vi "test enum2.vi"() -> ()   [LabVIEW 2020]
uses:
  OneDrive/_WorkingOn/Transformer-Project/Transformer/instr.lib/Ossila-X200-SMU-Driver/Public/Typedef/SMU OSR.ctl
  482ffdba-febc-40e4-8491-b362d5e89764.vi
  <userlib>/_NEVSTOP/Communicable State Machine(CSM)/addons/API-String-Arugments-Support/_Support/Convert API String Arguments to Data(variant).vi
  OneDrive/_WorkingOn/Transformer-Project/Transformer/instr.lib/Ossila-X200-SMU-Driver/Ossila X200 SMU.lvclass
panel:
  out "data 2":T1=enum."32768"
  out "Data":T1=enum."32768"
  out "data":T1=enum."32768"
  in  "element":string="4096"
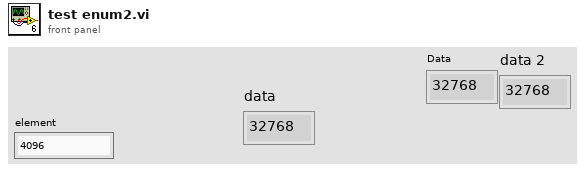
[diagram p1: front panel]
types:
  T1 = typedef "Ossila X200 SMU Instr.lvlib/Ossila X200 SMU.lvclass/SMU OSR.ctl" = enum16{"128", "256", "512", "1024", "2048", "4096", "8192", "16384", "32768"}
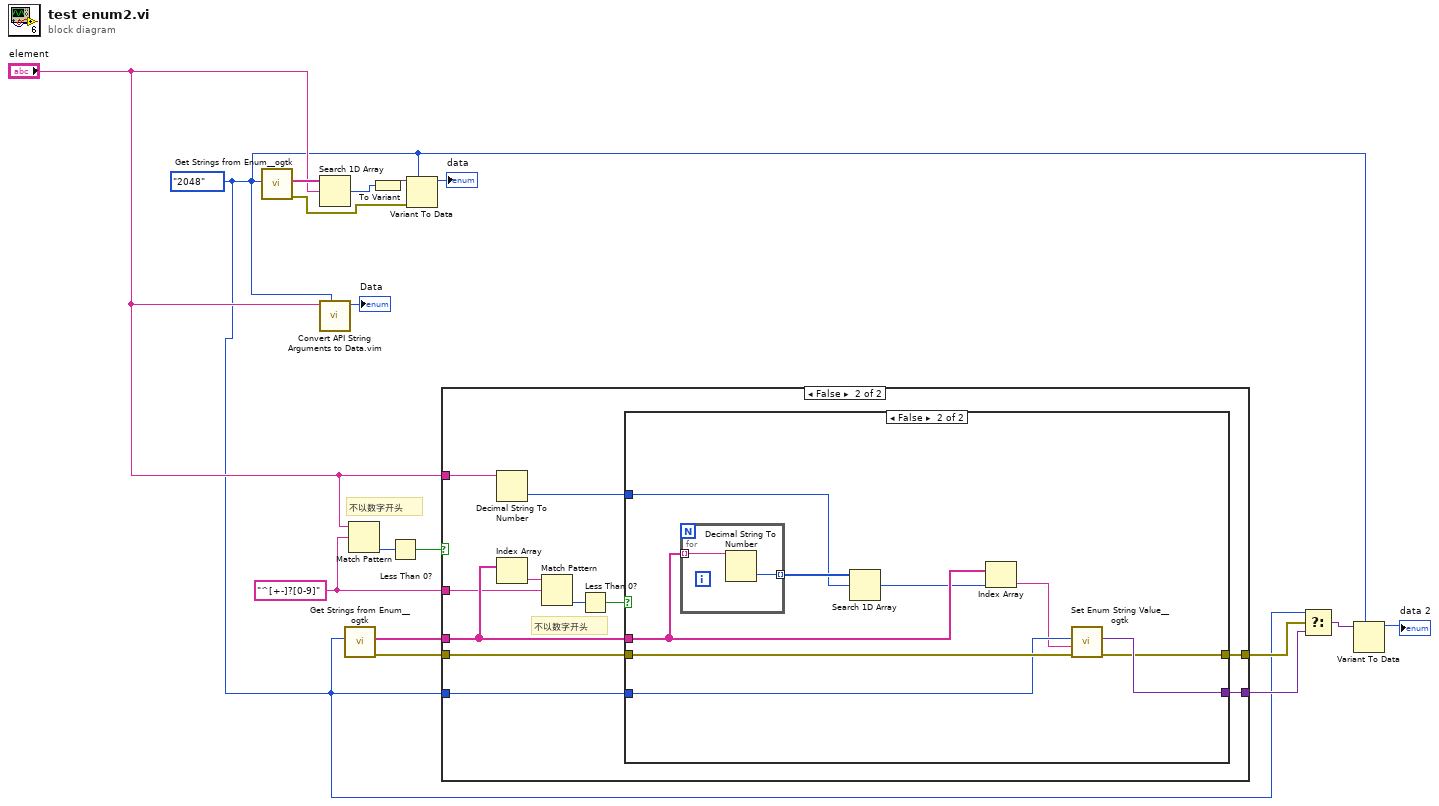
[diagram p0: block diagram]
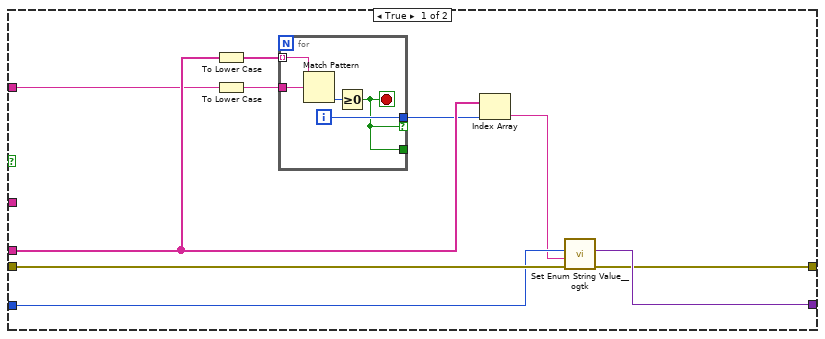
[diagram p2: hidden frame]
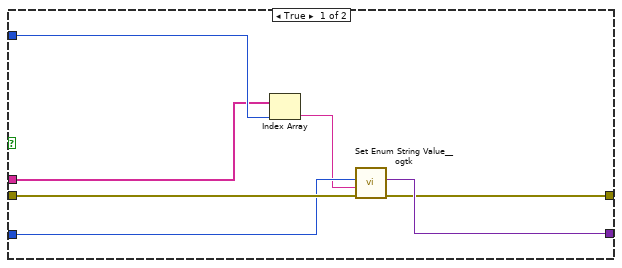
[diagram p3: hidden frame]
diagram:
  w6 = "^[+-]?[0-9]" ("regular expression")
  w2 = SMU_OSR."2048" ("OSR In")
  # "不以数字开头"
  n1 = call <userlib>:"Get Strings from Enum__ogtk.vi"("Enum"=w2) -> ("error out"=w14:errorcluster, "Enum Strings"=w17:string[])  [unwired: 7 in, 2 out]
  n2 = Search 1D Array(1D array=w17, element="element") -> (index of element=w15:i32)  [unwired: 1 in]
  n3 = call "Convert API String Arguments to Data.vim"("Type"=w2, "String"="element") -> ("Data"=→"Data":T1)  [unwired: 6 in, 1 out]
  n4 = call <userlib>:"Get Strings from Enum__ogtk.vi"("Enum"=w2) -> ("error out"=w10:errorcluster, "Enum Strings"=w9:string[])  [unwired: 7 in, 2 out]
  n5 = Match Pattern(string="element", regular expression=w6) -> (offset past match=w8:i32)  [unwired: 1 in, 3 out]
  n6 = To Variant(anything=w15) -> (Variant=w16:variant)
  n7 = Less Than 0?(x=w8) -> (x < 0?=w7:bool)
  n8 = Variant To Data(error in=w14, type=w2, Variant=w16) -> (data=→"data":T1)  [unwired: 1 out]
  n9 = case shown="False" w7 {
    tunnel: [w27 w43] -> w5
    tunnel: w10 -> [w26 w42]
    tunnel: w2 -> [w25 w41]
    tunnel: [w24 w40] -> w4
    tunnel: w9 -> [w23 w38]
    tunnel: "element" -> [w20 w39]
    tunnel: w6 -> [_ w35]
    frame True {
      n10 = To Lower Case(string=w23) -> (all lower case string=w19:string[])
      n11 = To Lower Case(string=w20) -> (all lower case string=w18:string)
      n12 = for {
        tunnel: w19 -> [w32] mode=indexing
        tunnel: w18 -> [w31]
        tunnel: [w30] -> w22 if=w28
        tunnel: [w28] -> _
        i -> [w30]
        stop <- w28 stop-if-true
        n13 = Match Pattern(string=w32, regular expression=w31) -> (offset past match=w29:i32)  [unwired: 1 in, 3 out]
        n14 = Greater Or Equal To 0?(x=w29) -> (x >= 0?=w28:bool)
      }
      n15 = Index Array(array=w23, index=w22) -> (element=w21:string)
      n16 = call <userlib>:"Set Enum String Value__ogtk.vi"("error in (no error)"=w26, "String Value"=w21, "Default Enum Value"=w25) -> ("error out"=w24:errorcluster, "Enum"=w27:variant)  [unwired: 7 in]
    }
    frame False {
      # "不以数字开头"
      n17 = Decimal String To Number(string=w39) -> (number=w33:i32)  [unwired: 2 in, 1 out]
      n18 = Index Array(array=w38) -> (element=w36:string)  [unwired: 1 in]
      n19 = Match Pattern(string=w36, regular expression=w35) -> (offset past match=w37:i32)  [unwired: 1 in, 3 out]
      n20 = Less Than 0?(x=w37) -> (x < 0?=w34:bool)
      n21 = case shown="False" w34 {
        tunnel: [w50 w59] -> w43
        tunnel: w42 -> [w49 w58]
        tunnel: w41 -> [w48 w57]
        tunnel: [w47 w56] -> w40
        tunnel: w38 -> [w45 w55]
        tunnel: w33 -> [w46 w52]
        frame True {
          n22 = Index Array(array=w45, index=w46) -> (element=w44:string)
          n23 = call <userlib>:"Set Enum String Value__ogtk.vi"("error in (no error)"=w49, "String Value"=w44, "Default Enum Value"=w48) -> ("error out"=w47:errorcluster, "Enum"=w50:variant)  [unwired: 7 in]
        }
        frame False {
          n24 = for {
            tunnel: w55 -> [w61] mode=indexing
            tunnel: [w60] -> w53 mode=indexing
            n25 = Decimal String To Number(string=w61) -> (number=w60:i32)  [unwired: 2 in, 1 out]
          }
          n26 = Search 1D Array(1D array=w53, element=w52) -> (index of element=w51:i32)  [unwired: 1 in]
          n27 = Index Array(array=w55, index=w51) -> (element=w54:string)
          n28 = call <userlib>:"Set Enum String Value__ogtk.vi"("error in (no error)"=w58, "String Value"=w54, "Default Enum Value"=w57) -> ("error out"=w56:errorcluster, "Enum"=w59:variant)  [unwired: 7 in]
        }
      }
    }
  }
  n29 = Select(t=w2, s=w4, f=w5) -> (s? t:f=w3:variant)
  n30 = Variant To Data(type=w2, Variant=w3) -> (data=→"data 2":T1)  [unwired: 1 in, 1 out]
